vi "startHWError.vi"(8 "error in (no error)":errorcluster, 11 "AtomChipHWC in":refnum<class "AtomChipHWC.lvclass">) -> (0 "error out":errorcluster, 2 "error":bool, 3 "AtomChipHWC out":refnum<class "AtomChipHWC.lvclass">)   [LabVIEW 2009, in "Hardware.lvlib" / "HWControllers.lvlib" / "AtomChipHWC.lvclass"]
uses:
  AtomChipHWC.lvclass
  AtomChipHWC.lvclass/AtomChipHWC.ctl
  Channels/Digital/DigitalOutput.lvclass
  Channels/VoltOutput/AnalogOutput.lvclass
  Channels/DDSOutput/Generic/DDSOutput.lvclass
  Network Controllers/CameraNetworkController/CameraNetworkController.lvclass
  HWController.lvclass
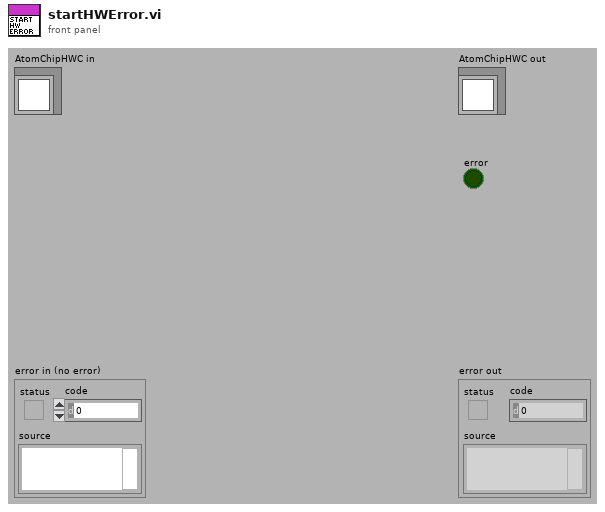
[diagram p1: front panel]
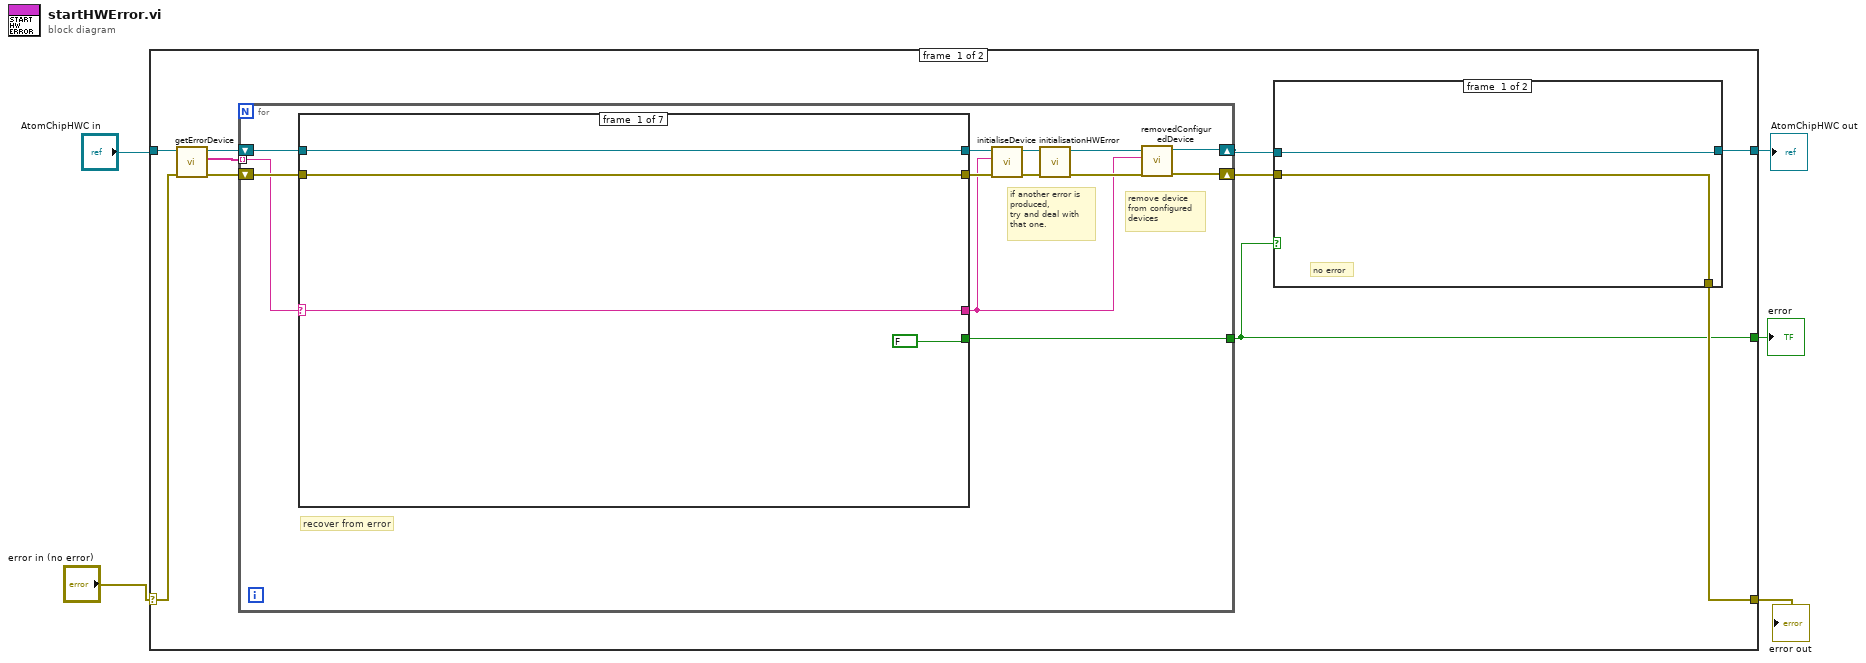
[diagram p0: block diagram]
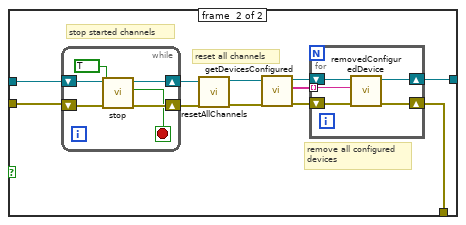
[diagram p2: hidden frame]
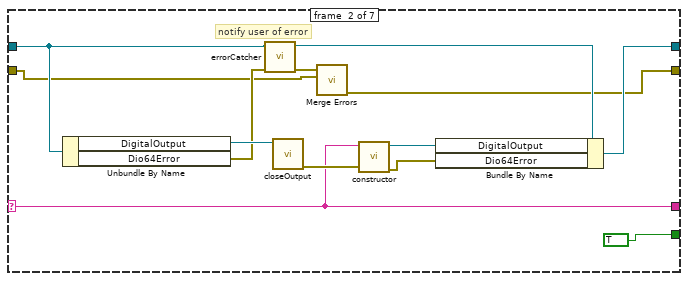
[diagram p3: hidden frame]
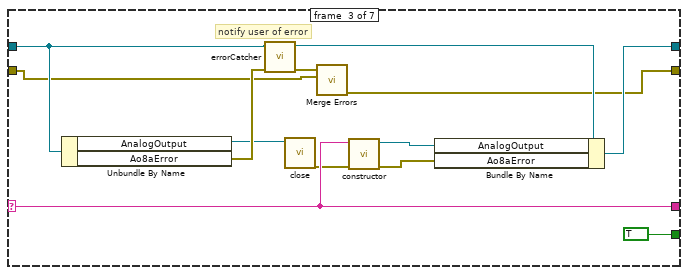
[diagram p4: hidden frame]
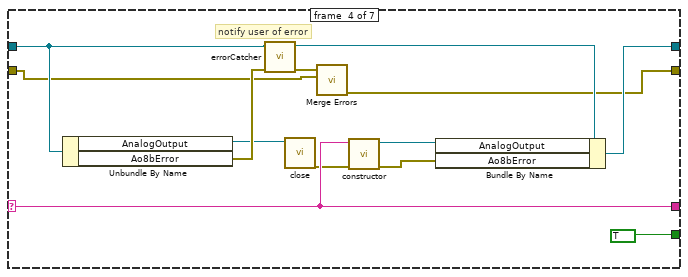
[diagram p5: hidden frame]
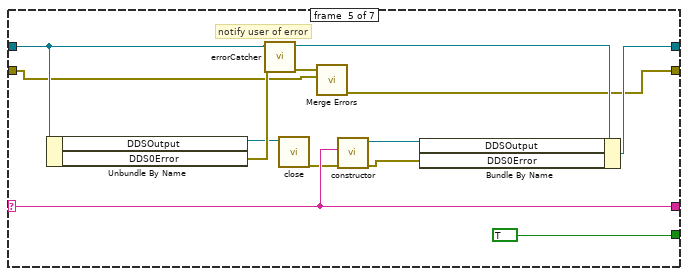
[diagram p6: hidden frame]
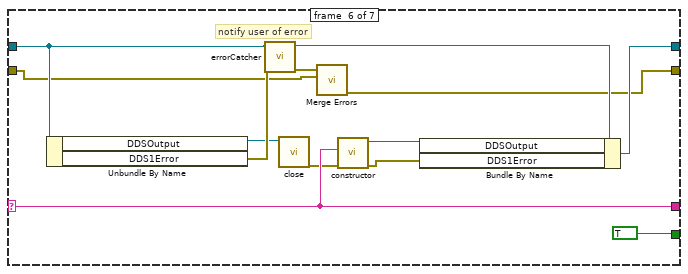
[diagram p7: hidden frame]
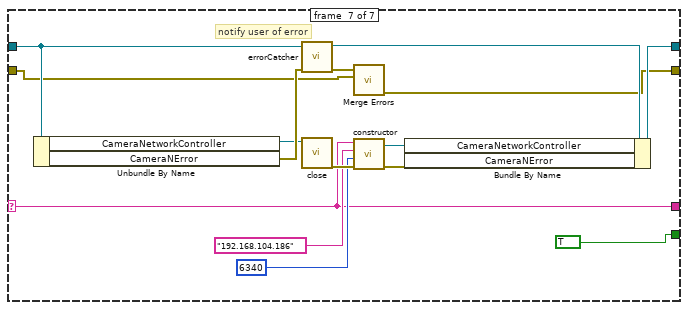
[diagram p8: hidden frame]
diagram:
  n1 = case shown="No Error" "error in (no error)" {
    selector: "error in (no error)" -> [w14 w137]
    tunnel: "AtomChipHWC in" -> [w15 w138]
    tunnel: [w9 w138] -> w2
    tunnel: [w10 w137] -> w3
    tunnel: [w6 _] -> w1
    frame #0 {
      n2 = call "getErrorDevice.vi"("error in (no error)"=w14, "AtomChipHWC in"=w15) -> ("error out"=w11:errorcluster, "Devices"=w12:string[], "AtomChipHWC out"=w13:refnum<class "AtomChipHWC.lvclass">)  [unwired: 7 in]
      n3 = for {
        tunnel: w12 -> [w50] mode=indexing
        shift-right: [w44] -> w8
        shift-left: w13 -> [w52]
        shift-right: [w43] -> w7
        shift-left: w11 -> [w51]
        tunnel: [w40] -> w6
        # "remove device\nfrom configured\ndevices"
        # "if another error is\nproduced,\ntry and deal with\nthat one."
        # "recover from error"
        n4 = case shown="\"Dio64\"" w50 {
          selector: w50 -> [w54 w58 w74 w87 w98 w111 w123]
          tunnel: w52 -> [w56 w65 w82 w95 w108 w121 w136]
          tunnel: [w56 w60 w77 w90 w103 w116 w131] -> w45
          tunnel: [w55 w59 w76 w89 w102 w115 w130] -> w42
          tunnel: w51 -> [w55 w61 w78 w91 w104 w117 w132]
          tunnel: [w54 w58 w74 w87 w98 w111 w123] -> w41
          tunnel: [FALSE TRUE TRUE TRUE TRUE TRUE TRUE] -> w40
          frame #0 {
          }
          frame #1 {
            # "notify user of error"
            n5 = Unbundle By Name(w65) -> ("DigitalOutput"=w69:refnum<class "DigitalOutput.lvclass">, "Dio64Error"=w63:errorcluster)
            n6 = call-dynamic "errorCatcher.vi"("error in (no error)"=w63, "HWController in"=w65) -> ("error out"=w62:errorcluster, "HWController out"=w64:refnum<class "AtomChipHWC.lvclass">)  [unwired: 8 in]
            n7 = call-dynamic "closeOutput.vi"("DigitalOutput in"=w69) -> ("error out"=w68:errorcluster)  [unwired: 10 in]
            n8 = call <vilib>:"Merge Errors.vi"("error in 2 (no error)"=w61, "error in 1 (no error)"=w62) -> ("error out"=w59:errorcluster)  [unwired: 5 in]
            n9 = call "constructor.vi"("error in (no error)"=w68, "deviceName"=w58) -> ("error out"=w66:errorcluster, "DigitalOutput out"=w67:refnum<class "DigitalOutput.lvclass">)  [unwired: 8 in]
            n10 = Bundle By Name(cluster=w64, "DigitalOutput"=w67, "Dio64Error"=w66) -> (w60:refnum<class "AtomChipHWC.lvclass">)
          }
          frame #2 {
            # "notify user of error"
            n11 = Unbundle By Name(w82) -> ("AnalogOutput"=w75:refnum<class "AnalogOutput.lvclass">, "Ao8aError"=w80:errorcluster)
            n12 = call-dynamic "errorCatcher.vi"("error in (no error)"=w80, "HWController in"=w82) -> ("error out"=w79:errorcluster, "HWController out"=w81:refnum<class "AtomChipHWC.lvclass">)  [unwired: 8 in]
            n13 = call-dynamic "close.vi"("AnalogOutput in"=w75) -> ("error out"=w73:errorcluster)  [unwired: 10 in]
            n14 = call <vilib>:"Merge Errors.vi"("error in 2 (no error)"=w78, "error in 1 (no error)"=w79) -> ("error out"=w76:errorcluster)  [unwired: 5 in]
            n15 = call "constructor.vi"("error in (no error)"=w73, "deviceName"=w74) -> ("error out"=w71:errorcluster, "AnalogOutput out"=w72:refnum<class "AnalogOutput.lvclass">)  [unwired: 8 in]
            n16 = Bundle By Name(cluster=w81, "AnalogOutput"=w72, "Ao8aError"=w71) -> (w77:refnum<class "AtomChipHWC.lvclass">)
          }
          frame #3 {
            # "notify user of error"
            n17 = Unbundle By Name(w95) -> ("AnalogOutput"=w88:refnum<class "AnalogOutput.lvclass">, "Ao8bError"=w93:errorcluster)
            n18 = call-dynamic "errorCatcher.vi"("error in (no error)"=w93, "HWController in"=w95) -> ("error out"=w92:errorcluster, "HWController out"=w94:refnum<class "AtomChipHWC.lvclass">)  [unwired: 8 in]
            n19 = call-dynamic "close.vi"("AnalogOutput in"=w88) -> ("error out"=w86:errorcluster)  [unwired: 10 in]
            n20 = call <vilib>:"Merge Errors.vi"("error in 2 (no error)"=w91, "error in 1 (no error)"=w92) -> ("error out"=w89:errorcluster)  [unwired: 5 in]
            n21 = call "constructor.vi"("error in (no error)"=w86, "deviceName"=w87) -> ("error out"=w84:errorcluster, "AnalogOutput out"=w85:refnum<class "AnalogOutput.lvclass">)  [unwired: 8 in]
            n22 = Bundle By Name(cluster=w94, "AnalogOutput"=w85, "Ao8bError"=w84) -> (w90:refnum<class "AtomChipHWC.lvclass">)
          }
          frame #4 {
            # "notify user of error"
            n23 = Unbundle By Name(w108) -> ("DDSOutput"=w101:refnum<class "DDSOutput.lvclass">, "DDS0Error"=w106:errorcluster)
            n24 = call-dynamic "errorCatcher.vi"("error in (no error)"=w106, "HWController in"=w108) -> ("error out"=w105:errorcluster, "HWController out"=w107:refnum<class "AtomChipHWC.lvclass">)  [unwired: 8 in]
            n25 = call-dynamic "close.vi"("DDSOutput in"=w101) -> ("error out"=w97:errorcluster)  [unwired: 10 in]
            n26 = call <vilib>:"Merge Errors.vi"("error in 2 (no error)"=w104, "error in 1 (no error)"=w105) -> ("error out"=w102:errorcluster)  [unwired: 5 in]
            n27 = call "constructor.vi"("error in (no error)"=w97, "device"=w98) -> ("error out"=w99:errorcluster, "DDSOutput out"=w100:refnum<class "DDSOutput.lvclass">)  [unwired: 8 in]
            n28 = Bundle By Name(cluster=w107, "DDSOutput"=w100, "DDS0Error"=w99) -> (w103:refnum<class "AtomChipHWC.lvclass">)
          }
          frame #5 {
            # "notify user of error"
            n29 = Unbundle By Name(w121) -> ("DDSOutput"=w114:refnum<class "DDSOutput.lvclass">, "DDS1Error"=w119:errorcluster)
            n30 = call-dynamic "errorCatcher.vi"("error in (no error)"=w119, "HWController in"=w121) -> ("error out"=w118:errorcluster, "HWController out"=w120:refnum<class "AtomChipHWC.lvclass">)  [unwired: 8 in]
            n31 = call-dynamic "close.vi"("DDSOutput in"=w114) -> ("error out"=w110:errorcluster)  [unwired: 10 in]
            n32 = call <vilib>:"Merge Errors.vi"("error in 2 (no error)"=w117, "error in 1 (no error)"=w118) -> ("error out"=w115:errorcluster)  [unwired: 5 in]
            n33 = call "constructor.vi"("error in (no error)"=w110, "device"=w111) -> ("error out"=w112:errorcluster, "DDSOutput out"=w113:refnum<class "DDSOutput.lvclass">)  [unwired: 8 in]
            n34 = Bundle By Name(cluster=w120, "DDSOutput"=w113, "DDS1Error"=w112) -> (w116:refnum<class "AtomChipHWC.lvclass">)
          }
          frame #6 {
            # "notify user of error"
            n35 = Unbundle By Name(w136) -> ("CameraNetworkController"=w129:refnum<class "CameraNetworkController.lvclass">, "CameraNError"=w134:errorcluster)
            n36 = call-dynamic "errorCatcher.vi"("error in (no error)"=w134, "HWController in"=w136) -> ("error out"=w133:errorcluster, "HWController out"=w135:refnum<class "AtomChipHWC.lvclass">)  [unwired: 8 in]
            n37 = call "close.vi"("CameraNetworkController in"=w129) -> ("error out"=w126:errorcluster)  [unwired: 9 in, 1 out]
            n38 = call <vilib>:"Merge Errors.vi"("error in 2 (no error)"=w132, "error in 1 (no error)"=w133) -> ("error out"=w130:errorcluster)  [unwired: 5 in]
            n39 = call "constructor.vi"("error in (no error)"=w126, "remote port"=u16 6340, "remote address"="192.168.104.186", "camera"=w123) -> ("error out"=w127:errorcluster, "CameraNetworkController out"=w128:refnum<class "CameraNetworkController.lvclass">)  [unwired: 6 in]
            n40 = Bundle By Name(cluster=w135, "CameraNetworkController"=w128, "CameraNError"=w127) -> (w131:refnum<class "AtomChipHWC.lvclass">)
          }
        }
        n41 = call "initialiseDevice.vi"("error in (no error)"=w42, "deviceName"=w41, "AtomChipHWC in"=w45) -> ("error out"=w48:errorcluster, "AtomChipHWC out"=w49:refnum<class "AtomChipHWC.lvclass">)  [unwired: 7 in]
        n42 = call-dynamic "initialisationHWError.vi"("error in (no error)"=w48, "AtomChipHWC in"=w49) -> ("error out"=w46:errorcluster, "AtomChipHWC out"=w47:refnum<class "AtomChipHWC.lvclass">)  [unwired: 8 in]
        n43 = call-dynamic "removedConfiguredDevice.vi"("error in (no error)"=w46, "device"=w41, "HWController in"=w47) -> ("error out"=w43:errorcluster, "HWController out"=w44:refnum<class "AtomChipHWC.lvclass">)  [unwired: 7 in]
      }
      n44 = case shown="True" w6 {
        tunnel: [w16 w24] -> w10
        tunnel: [w17 w23] -> w9
        tunnel: w8 -> [w17 w21]
        tunnel: w7 -> [w16 w20]
        frame #0 {
          # "no error"
        }
        frame #1 {
          # "stop started channels"
          # "remove all configured\ndevices"
          # "reset all channels"
          n45 = while {
            shift-right: [w32] -> w19
            shift-left: w21 -> [w34]
            shift-right: [w31] -> w18
            shift-left: w20 -> [w33]
            stop <- w30 stop-if-true
            n46 = call-dynamic "stop.vi"("error in (no error)"=w33, "stop?"=TRUE, "AtomChipHWC in"=w34) -> ("error out"=w31:errorcluster, "stopped"=w30:bool, "AtomChipHWC out"=w32:refnum<class "AtomChipHWC.lvclass">)  [unwired: 6 in]
          }
          n47 = call-dynamic "resetAllChannels.vi"("error in (no error)"=w18, "AtomChipHWC in"=w19) -> ("error out"=w27:errorcluster, "AtomChipHWC out"=w28:refnum<class "AtomChipHWC.lvclass">)  [unwired: 8 in]
          n48 = call "getDevicesConfigured.vi"("error in (no error)"=w27, "HWController.lvclass in"=w28) -> ("error out"=w25:errorcluster, "devicesConfigured"=w22:string[], "HWController.lvclass out"=w26:refnum<class "AtomChipHWC.lvclass">)  [unwired: 7 in]
          n49 = for {
            shift-right: [w38] -> w23
            shift-left: w26 -> [w39]
            shift-right: [w36] -> w24
            shift-left: w25 -> [w37]
            tunnel: w22 -> [w35] mode=indexing
            n50 = call-dynamic "removedConfiguredDevice.vi"("error in (no error)"=w37, "device"=w35, "HWController in"=w39) -> ("error out"=w36:errorcluster, "HWController out"=w38:refnum<class "AtomChipHWC.lvclass">)  [unwired: 7 in]
          }
        }
      }
    }
    frame #1 {
    }
  }
  "error out" <- w3
  "AtomChipHWC out" <- w2
  "error" <- w1
